vi "Advance past Number.vi"(7 "JSON":string, 9 "Offset (0)":i32, 11 "Parser State in":T2=enum."Number/Other") -> (1 "Offset past match":i32, 3 "Parser State":T2, 4 "JSON Value Type":T1, 6 "Value start out":i32)   [LabVIEW 2017, in "JSONtext.lvlib"]
uses:
  JSONtext.lvlib
  Parsing State.ctl
  JSON Value Type.ctl
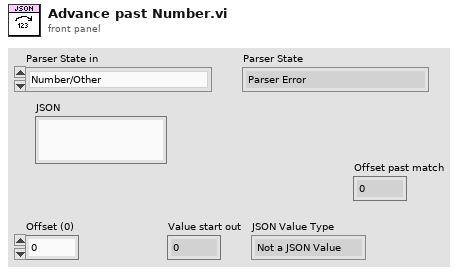
[diagram p1: front panel]
types:
  T1 = typedef "JSONtext.lvlib/JSON Value Type.ctl" = enum16{"Not a JSON Value", "JSON Object", "JSON Array", "String", "Number", "true", "false", "null"}
  T2 = typedef "JSONtext.lvlib/Parsing State.ctl" = enum16{"Parser Error", "Object", "Array", "String", "Number/Other", "Leading Whitespace", "Object end", "Array end", "Value end"}
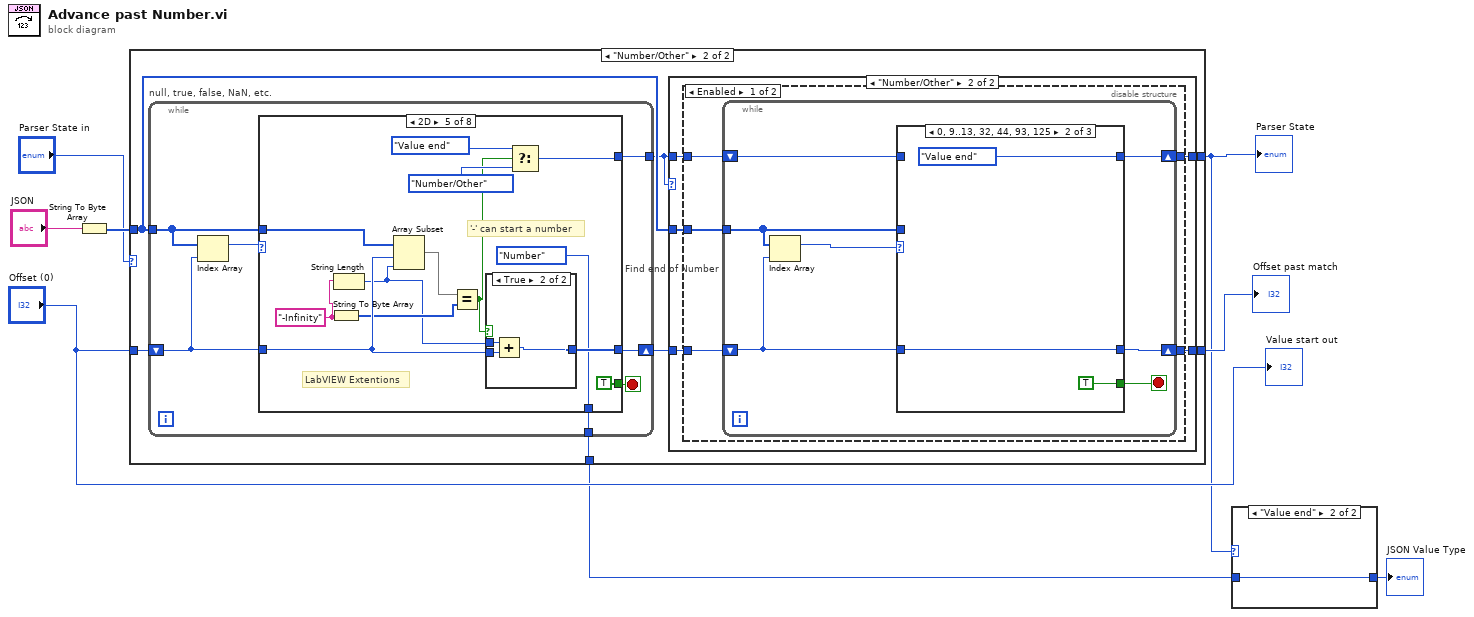
[diagram p0: block diagram]
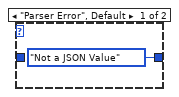
[diagram p2: hidden frame]
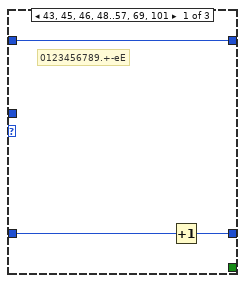
[diagram p5: hidden frame]
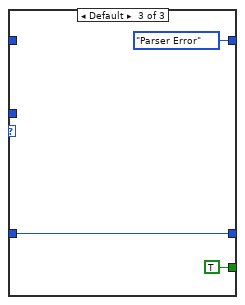
[diagram p6: hidden frame]
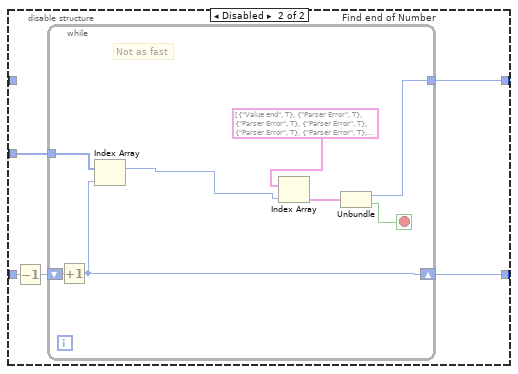
[diagram p7: hidden frame]
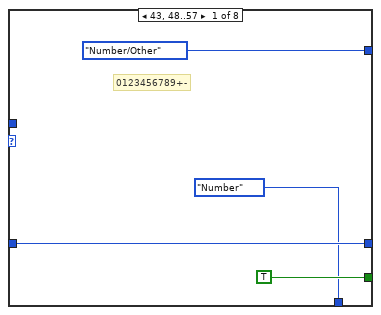
[diagram p8: hidden frame]
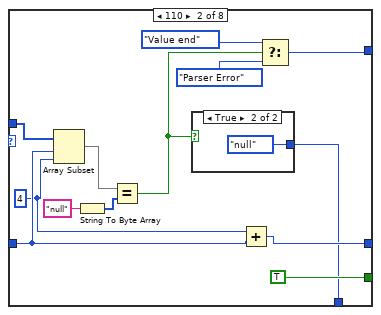
[diagram p9: hidden frame]
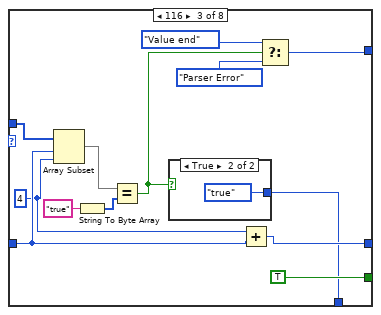
[diagram p11: hidden frame]
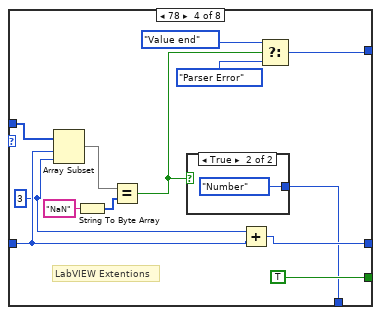
[diagram p13: hidden frame]
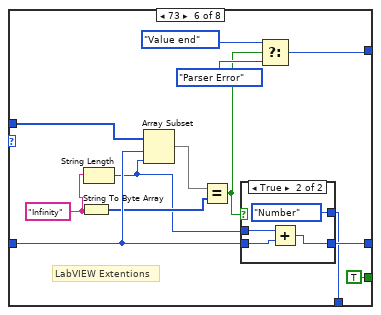
[diagram p16: hidden frame]
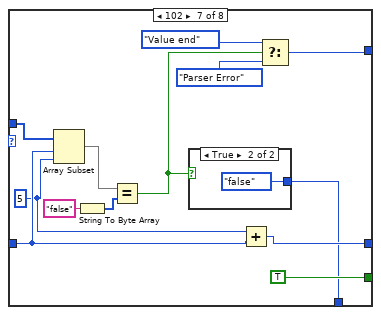
[diagram p18: hidden frame]
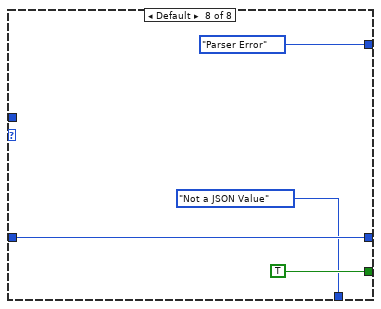
[diagram p20: hidden frame]
diagram:
  n1 = String To Byte Array(string="JSON") -> (unsigned byte array=w5:u8[])
  n2 = case shown="\"Number/Other\"" "Parser State in" {
    tunnel: [_ w16] -> w3
    tunnel: [w9 w15] -> w8
    tunnel: w5 -> [_ w13]
    tunnel: "Offset (0)" -> [w9 w11]
    tunnel: [_ w10] -> w2
    frame "Parser Error", Default {
    }
    frame "Number/Other" {
      n3 = while "null, true, false, NaN, etc." {
        tunnel: w13 -> [w63]
        shift-right: [w59] -> w14
        shift-left: w11 -> [w60]
        tunnel: [w62] -> w12
        tunnel: [w58] -> w10
        stop <- w61 stop-if-true
        n4 = Index Array(array=w63, index=w60) -> (element=w64:u8)
        n5 = case shown="2D" w64 {
          tunnel: w63 -> [_ w80 w94 w108 w123 w140 w157 _]
          tunnel: [Parsing_State."Number/Other" w77 w91 w105 w121 w138 w154 Parsing_State."Parser Error"] -> w62
          tunnel: [TRUE TRUE TRUE TRUE TRUE TRUE TRUE TRUE] -> w61
          tunnel: w60 -> [w66 w73 w87 w101 w117 w134 w150 w163]
          tunnel: [w66 w71 w85 w99 w116 w133 w148 w163] -> w59
          tunnel: [JSON_Value_Type."Number" w69 w83 w97 JSON_Value_Type."Number" w128 w146 JSON_Value_Type."Not a JSON Value"] -> w58
          frame 43, 48..57 {
            # "0123456789+-"
          }
          frame 110 {
            w72 = 4 ("length")
            n6 = Array Subset(array=w80, index=w73, length=w72) -> (w78:u8[])
            n7 = String To Byte Array(string="null") -> (unsigned byte array=w79:u8[])
            n8 = Equal?(x=w78, y=w79) -> (x = y?=w70:bool)
            n9 = case shown="True" w70 {
              tunnel: [_ JSON_Value_Type."null"] -> w69
              frame False {
              }
              frame True {
              }
            }
            n10 = Add(x=w72, y=w73) -> (x+y=w71:i32)
            n11 = Select(t=Parsing_State."Value end", s=w70, f=Parsing_State."Parser Error") -> (s? t:f=w77:T2)
          }
          frame 116 {
            w86 = 4 ("length")
            n12 = Array Subset(array=w94, index=w87, length=w86) -> (w92:u8[])
            n13 = String To Byte Array(string="true") -> (unsigned byte array=w93:u8[])
            n14 = Equal?(x=w92, y=w93) -> (x = y?=w84:bool)
            n15 = case shown="True" w84 {
              tunnel: [_ JSON_Value_Type."true"] -> w83
              frame False {
              }
              frame True {
              }
            }
            n16 = Add(x=w86, y=w87) -> (x+y=w85:i32)
            n17 = Select(t=Parsing_State."Value end", s=w84, f=Parsing_State."Parser Error") -> (s? t:f=w91:T2)
          }
          frame 78 {
            w100 = 3 ("length")
            # "LabVIEW Extentions"
            n18 = Array Subset(array=w108, index=w101, length=w100) -> (w106:u8[])
            n19 = String To Byte Array(string="NaN") -> (unsigned byte array=w107:u8[])
            n20 = Equal?(x=w106, y=w107) -> (x = y?=w98:bool)
            n21 = case shown="True" w98 {
              tunnel: [_ JSON_Value_Type."Number"] -> w97
              frame False {
              }
              frame True {
              }
            }
            n22 = Add(x=w100, y=w101) -> (x+y=w99:i32)
            n23 = Select(t=Parsing_State."Value end", s=w98, f=Parsing_State."Parser Error") -> (s? t:f=w105:T2)
          }
          frame 45 {
            w114 = "-Infinity"
            # "'-' can start a number"
            # "LabVIEW Extentions"
            n24 = String To Byte Array(string=w114) -> (unsigned byte array=w115:u8[])
            n25 = String Length(string=w114) -> (length=w113:i32)
            n26 = Array Subset(array=w123, index=w117, length=w113) -> (w122:u8[])
            n27 = Equal?(x=w122, y=w115) -> (x = y?=w112:bool)
            n28 = case shown="True" w112 {
              tunnel: w117 -> [w124 w127]
              tunnel: [w124 w126] -> w116
              tunnel: w113 -> [_ w125]
              frame False {
              }
              frame True {
                n29 = Add(x=w125, y=w127) -> (x+y=w126:i32)
              }
            }
            n30 = Select(t=Parsing_State."Value end", s=w112, f=Parsing_State."Number/Other") -> (s? t:f=w121:T2)
          }
          frame 73 {
            w131 = "Infinity"
            # "LabVIEW Extentions"
            n31 = String To Byte Array(string=w131) -> (unsigned byte array=w132:u8[])
            n32 = String Length(string=w131) -> (length=w130:i32)
            n33 = Array Subset(array=w140, index=w134, length=w130) -> (w139:u8[])
            n34 = Equal?(x=w139, y=w132) -> (x = y?=w129:bool)
            n35 = case shown="True" w129 {
              tunnel: w134 -> [w141 w145]
              tunnel: [w141 w144] -> w133
              tunnel: w130 -> [_ w143]
              tunnel: [_ JSON_Value_Type."Number"] -> w128
              frame False {
              }
              frame True {
                n36 = Add(x=w143, y=w145) -> (x+y=w144:i32)
              }
            }
            n37 = Select(t=Parsing_State."Value end", s=w129, f=Parsing_State."Parser Error") -> (s? t:f=w138:T2)
          }
          frame 102 {
            w149 = 5 ("length")
            n38 = Array Subset(array=w157, index=w150, length=w149) -> (w155:u8[])
            n39 = String To Byte Array(string="false") -> (unsigned byte array=w156:u8[])
            n40 = Equal?(x=w155, y=w156) -> (x = y?=w147:bool)
            n41 = case shown="True" w147 {
              tunnel: [_ JSON_Value_Type."false"] -> w146
              frame False {
              }
              frame True {
              }
            }
            n42 = Add(x=w149, y=w150) -> (x+y=w148:i32)
            n43 = Select(t=Parsing_State."Value end", s=w147, f=Parsing_State."Parser Error") -> (s? t:f=w154:T2)
          }
          frame Default {
          }
        }
      }
      n44 = case shown="\"Number/Other\"" w12 {
        tunnel: [w17 w23] -> w16
        tunnel: [w18 w22] -> w15
        tunnel: w14 -> [w18 w19]
        tunnel: w12 -> [w17 w21]
        tunnel: w13 -> [_ w20]
        frame "Parser Error", Default {
        }
        frame "Number/Other" {
          n45 = disable-structure shown="Enabled" {
            disable-tunnel: [w28 w49] -> w23
            disable-tunnel: [w27 w48] -> w22
            disable-tunnel: w21 -> [w26 _]
            disable-tunnel: w20 -> [w25 w47]
            disable-tunnel: w19 -> [w24 w46]
            frame Enabled {
              n46 = while "Find end of Number" {
                tunnel: w25 -> [w35]
                shift-right: [w31] -> w27
                shift-left: w24 -> [w29]
                shift-right: [w33] -> w28
                shift-left: w26 -> [w34]
                stop <- w32 stop-if-true
                n47 = Index Array(array=w35, index=w29) -> (element=w30:u8)
                n48 = case shown="0, 9..13, 32, 44, 93, 125" w30 {
                  tunnel: w35 -> [_ _ _]
                  tunnel: w34 -> [w38 _ _]
                  tunnel: [w38 Parsing_State."Value end" Parsing_State."Parser Error"] -> w33
                  tunnel: [_ TRUE TRUE] -> w32
                  tunnel: w29 -> [w37 w39 w44]
                  tunnel: [w36 w39 w44] -> w31
                  frame 43, 45, 46, 48..57, 69, 101 {
                    # "0123456789.+-eE"
                    n49 = Increment(x=w37) -> (x+1=w36:i32)
                  }
                  frame 0, 9..13, 32, 44, 93, 125 {
                  }
                  frame Default {
                  }
                }
              }
            }
            frame Disabled {
              n50 = Decrement(x=w46) -> (x-1=w45:i32)
              n51 = while "Find end of Number" {
                tunnel: w47 -> [w57]
                shift-right: [w50] -> w48
                shift-left: w45 -> [w56]
                tunnel: [w51] -> w49
                stop <- w52 stop-if-true
                # "Not as fast"
                n52 = Increment(x=w56) -> (x+1=w50:i32)
                n53 = Index Array(array=w57, index=w50) -> (element=w53:u8)
                n54 = Index Array(array=cluster{T2, bool}[] [{enum."Value end", TRUE}, {enum."Parser Error", TRUE}, {enum."Parser Error", TRUE}, {enum."Parser Error", TRUE}, {enum."Parser Error", TRUE}, {enum."Parser Error", TRUE}, {enum."Parser Error", TRUE}, {enum."Parser Error", TRUE}, {enum."Parser Error", TRUE}, {enum."Value end", TRUE}, {enum."Value end", TRUE}, {enum."Value end", TRUE}, {enum."Value end", TRUE}, {enum."Value end", TRUE}, {enum."Parser Error", TRUE}, {enum."Parser Error", TRUE}, {enum."Parser Error", TRUE}, {enum."Parser Error", TRUE}, {enum."Parser Error", TRUE}, {enum."Parser Error", TRUE}, {enum."Parser Error", TRUE}, {enum."Parser Error", TRUE}, {enum."Parser Error", TRUE}, {enum."Parser Error", TRUE}, {enum."Parser Error", TRUE}, {enum."Parser Error", TRUE}, {enum."Parser Error", TRUE}, {enum."Parser Error", TRUE}, {enum."Parser Error", TRUE}, {enum."Parser Error", TRUE}, {enum."Parser Error", TRUE}, {enum."Parser Error", TRUE}, {enum."Value end", TRUE}, {enum."Parser Error", TRUE}, {enum."Parser Error", TRUE}, {enum."Parser Error", TRUE}, {enum."Parser Error", TRUE}, {enum."Parser Error", TRUE}, {enum."Parser Error", TRUE}, {enum."Parser Error", TRUE}, {enum."Parser Error", TRUE}, {enum."Parser Error", TRUE}, {enum."Parser Error", TRUE}, {enum."Number/Other", FALSE}, {enum."Value end", TRUE}, {enum."Number/Other", FALSE}, {enum."Number/Other", FALSE}, {enum."Parser Error", TRUE}, {enum."Number/Other", FALSE}, {enum."Number/Other", FALSE}, {enum."Number/Other", FALSE}, {enum."Number/Other", FALSE}, {enum."Number/Other", FALSE}, {enum."Number/Other", FALSE}, {enum."Number/Other", FALSE}, {enum."Number/Other", FALSE}, {enum."Number/Other", FALSE}, {enum."Number/Other", FALSE}, {enum."Parser Error", TRUE}, {enum."Parser Error", TRUE}, {enum."Parser Error", TRUE}, {enum."Parser Error", TRUE}, {enum."Parser Error", TRUE}, {enum."Parser Error", TRUE}, {enum."Parser Error", TRUE}, {enum."Parser Error", TRUE}, {enum."Parser Error", TRUE}, {enum."Parser Error", TRUE}, {enum."Parser Error", TRUE}, {enum."Number/Other", FALSE}, {enum."Parser Error", TRUE}, {enum."Parser Error", TRUE}, {enum."Parser Error", TRUE}, {enum."Parser Error", TRUE}, {enum."Parser Error", TRUE}, {enum."Parser Error", TRUE}, {enum."Parser Error", TRUE}, {enum."Parser Error", TRUE}, {enum."Parser Error", TRUE}, {enum."Parser Error", TRUE}, {enum."Parser Error", TRUE}, {enum."Parser Error", TRUE}, {enum."Parser Error", TRUE}, {enum."Parser Error", TRUE}, {enum."Parser Error", TRUE}, {enum."Parser Error", TRUE}, {enum."Parser Error", TRUE}, {enum."Parser Error", TRUE}, {enum."Parser Error", TRUE}, {enum."Parser Error", TRUE}, {enum."Parser Error", TRUE}, {enum."Parser Error", TRUE}, {enum."Parser Error", TRUE}, {enum."Value end", TRUE}, {enum."Parser Error", TRUE}, {enum."Parser Error", TRUE}, {enum."Parser Error", TRUE}, {enum."Parser Error", TRUE}, {enum."Parser Error", TRUE}, {enum."Parser Error", TRUE}, {enum."Parser Error", TRUE}, {enum."Number/Other", FALSE}, {enum."Parser Error", TRUE}, {enum."Parser Error", TRUE}, {enum."Parser Error", TRUE}, {enum."Parser Error", TRUE}, {enum."Parser Error", TRUE}, {enum."Parser Error", TRUE}, {enum."Parser Error", TRUE}, {enum."Parser Error", TRUE}, {enum."Parser Error", TRUE}, {enum."Parser Error", TRUE}, {enum."Parser Error", TRUE}, {enum."Parser Error", TRUE}, {enum."Parser Error", TRUE}, {enum."Parser Error", TRUE}, {enum."Parser Error", TRUE}, {enum."Parser Error", TRUE}, {enum."Parser Error", TRUE}, {enum."Parser Error", TRUE}, {enum."Parser Error", TRUE}, {enum."Parser Error", TRUE}, {enum."Parser Error", TRUE}, {enum."Parser Error", TRUE}, {enum."Parser Error", TRUE}, {enum."Value end", TRUE}] ("Array"), index=w53) -> (element=w54:cluster{T2, bool})
                n55 = Unbundle(w54) -> (w51:T2, w52:bool)
              }
            }
          }
        }
      }
    }
  }
  "Parser State" <- w3
  "Offset past match" <- w8
  n56 = case shown="\"Value end\"" w3 {
    tunnel: w2 -> [_ w165]
    tunnel: [JSON_Value_Type."Not a JSON Value" w165] -> w1
    frame "Parser Error", Default {
    }
    frame "Value end" {
    }
  }
  "JSON Value Type" <- w1
  "Value start out" <- "Offset (0)"
